vi "OpenFile.vi"(8 "error in (no error)":errorcluster, 10 "File Path":path) -> (0 "error out":errorcluster, 3 "ROFile out":refnum<class "ROFile.lvclass">)   [LabVIEW 2021, in "ROFile.lvclass"]
uses:
  ROFile.lvclass
  ROFile.lvclass/ROFile.ctl
  File/File.lvclass
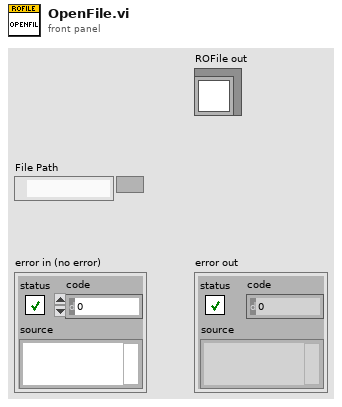
[diagram p1: front panel]
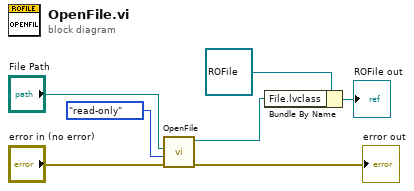
[diagram p0: block diagram]
diagram:
  n1 = call "OpenFile.vi"("error in (no error)"="error in (no error)", "access (0:read/write)"=enum16{"read/write", "read-only", "write-only"}."read-only", "File Path"="File Path") -> ("error out"=→"error out":errorcluster, "File out"=w1:refnum<class "File.lvclass">)  [unwired: 7 in]
  n2 = Bundle By Name(cluster=refnum<class "ROFile.lvclass"> refnum ("ROFile in"), "File.lvclass"=w1) -> (→"ROFile out":refnum<class "ROFile.lvclass">)
